vi "Drivetrain Manager.vi"(10 "setpoint":dbl) -> ()   [LabVIEW 2014]
uses:
  Robot Global Data.vi
  <vilib>/Rock Robotics/WPI/RobotDrive/WPI_RobotDriveGetSetRefNum.vi
  <vilib>/addons/control/pid/NI_PID_pid.lvlib
  <vilib>/addons/control/pid/pid.llb/PID (DBL).vi
panel:
  in  "PID gains":T1={"proportional gain (Kc)"=1.0, "integral time (Ti, min)"=0.01, "derivative time (Td, min)"=0.0} {"derivative time (Td, min)" format="%.3f"; "integral time (Ti, min)" format="%.3f"; "proportional gain (Kc)" format="%.3f"}
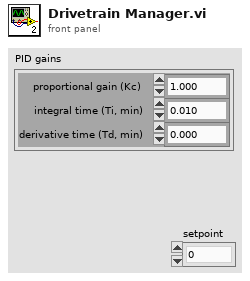
[diagram p1: front panel]
types:
  T1 = cluster{"proportional gain (Kc)":dbl, "integral time (Ti, min)":dbl, "derivative time (Td, min)":dbl}
  T2 = typedef "WPI_EncoderDevRef.ctl" = cluster{"DevStatus":errorcluster, "EncoderIndex":T3, "CounterIndex":T4, "DistancePerCount":dbl, "Decoding Type":T5}
  T3 = typedef "FPGA_EncoderIdx.ctl" = enum8{"Enc 0", "Enc 1", "Enc 2", "Enc 3", "Enc 4", "Enc 5", "Enc 6", "Enc 7", "Invalid"}
  T4 = typedef "FPGA_CounterCtrSystemIndex.ctl" = enum8{"Ctr 0", "Ctr 1", "Ctr 2", "Ctr 3", "Ctr 4", "Ctr 5", "Ctr 6", "Ctr 7", "Invalid"}
  T5 = typedef "WPI_EncoderType.ctl" = enum16{"1x", "2x", "4x"}
  T6 = typedef "WPI_RobotDriveDevRef.ctl" = cluster{"DevStatus":errorcluster, "Motors[]":T7[], "Square Inputs":bool, "Max Output":dbl}
  T7 = typedef "WPI_MotorControlDeviceRef.ctl" = cluster{"DeviceStatus":errorcluster, "Type":T8, "PWM":cluster{"Controller":T9, "PWM Channel":T10, "DeadBand":T11}, "CAN":cluster{"Device Number":u8, "Control Mode":T12, "Semaphore":T13, "Max Vout":dbl, "TalonSRX Control Mode":T14}, "Invert":bool, "TransformRef":T15, "InvTransformRef":T15}
  T8 = typedef "WPI_MotorControlType.ctl" = enum16{"PWM", "CAN", "CANTalonSRX"}
  T9 = typedef "FPGA_TypedefDigitalModule.ctl" = enum16{"Controller 1"}
  T10 = typedef "FPGA_DIOPWMChannel.ctl" = enum8{"PWM 0", "PWM 1", "PWM 2", "PWM 3", "PWM 4", "PWM 5", "PWM 6", "PWM 7", "PWM 8", "PWM 9", "PWM MXP 0", "PWM MXP 1", "PWM MXP 2", "PWM MXP 3", "PWM MXP 4", "PWM MXP 5", "PWM MXP 6", "PWM MXP 7", "PWM MXP 8", "PWM MXP 9", "Invalid"}
  T11 = typedef "WPI_PWMDeadband.ctl" = cluster{"Name":string, "maxPositivePwm":i32, "minPositivePwm":i32, "centerPwm":i32, "maxNegativePwm":i32, "minNegativePwm":i32, "angularRange":u16}
  T12 = typedef "WPI_CANJaguar_ControlMode.ctl" = enum8{"Percent VBus", "Current", "Speed", "Position", "Voltage"}
  T13 = typedef "Semaphore RefNum" = refnum<k1>
  T14 = typedef "WPI_CANTalonSRX_APIControlMode.ctl" = enum8{"Percent VBus", "Speed", "Position", "Slave", "Unchanged / Invalid"}
  T15 = typedef "WPI_PWMTransform_ConPane.ctl" = refnum<vi>
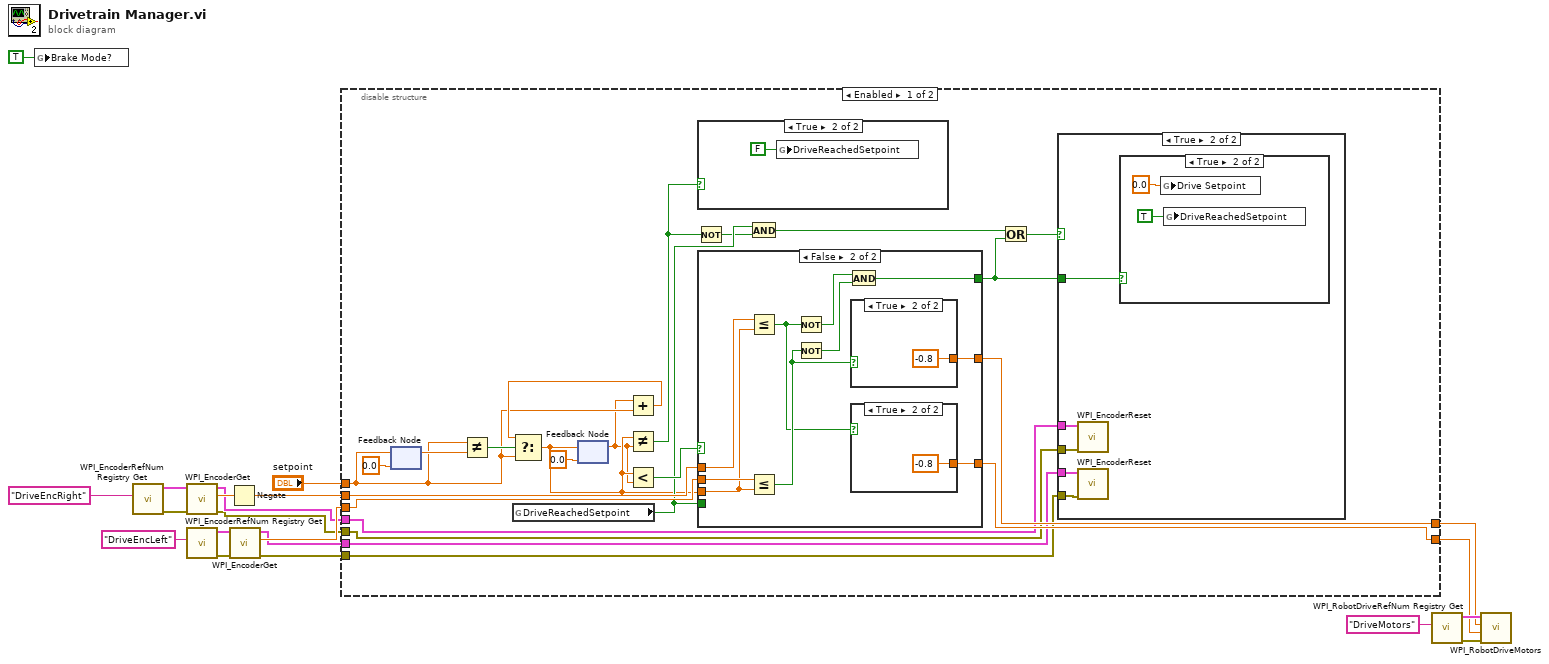
[diagram p0: block diagram]
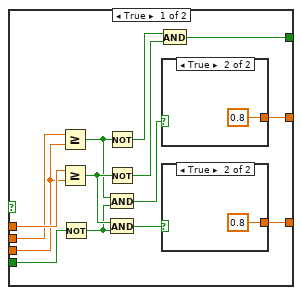
[diagram p5: hidden frame]
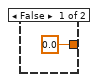
[diagram p6: hidden frame]
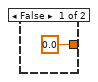
[diagram p7: hidden frame]
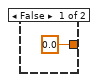
[diagram p8: hidden frame]
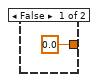
[diagram p9: hidden frame]
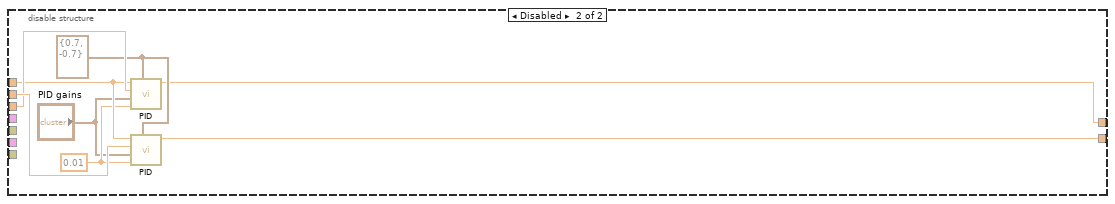
[diagram p10: hidden frame]
diagram:
  n1 = global write "Robot Global Data.vi" "Brake Mode?"(TRUE) -> ()
  n2 = call <vilib>:"WPI_EncoderRefNum Registry Get.vi"("refnum name"="DriveEncRight") -> ("error out"=w13:errorcluster, "EncoderDevRef"=w14:T2)  [unwired: 9 in]
  n3 = call <vilib>:"WPI_EncoderGet.vi"("error in (no error)"=w13, "EncoderDevRef"=w14) -> ("error out"=w1:errorcluster, "Distance"=w6:dbl, "EncoderDevRef"=w2:T2)  [unwired: 4 in, 3 out]
  n4 = call <vilib>:"WPI_EncoderRefNum Registry Get.vi"("refnum name"="DriveEncLeft") -> ("error out"=w10:errorcluster, "EncoderDevRef"=w11:T2)  [unwired: 9 in]
  n5 = Negate(x=w6) -> (-x=w5:dbl)
  n6 = call <vilib>:"WPI_EncoderGet.vi"("error in (no error)"=w10, "EncoderDevRef"=w11) -> ("error out"=w3:errorcluster, "Distance"=w7:dbl, "EncoderDevRef"=w4:T2)  [unwired: 4 in, 3 out]
  n7 = disable-structure shown="Enabled" {
    disable-tunnel: [w42 w85] -> w16
    disable-tunnel: [w41 w86] -> w15
    disable-tunnel: "setpoint" -> [w23 w89]
    disable-tunnel: w7 -> [w40 w90]
    disable-tunnel: w5 -> [w39 w91]
    disable-tunnel: w4 -> [w35 _]
    disable-tunnel: w3 -> [w36 _]
    disable-tunnel: w2 -> [w37 _]
    disable-tunnel: w1 -> [w38 _]
    frame Enabled {
      n8 = feedback #1(0.0 ("setpoint")) -> (w26:dbl)
      n9 = feedback-in #1(w23) -> ()
      n10 = Not Equal?(x=w23, y=w26) -> (x != y?=w25:bool)
      n11 = global read "Robot Global Data.vi" "DriveReachedSetpoint"() -> (w34:bool)
      n12 = feedback #2(0.0 ("setpoint")) -> (w21:dbl)
      n13 = Add(x=w21, y=w23) -> (x+y=w24:dbl)
      n14 = Select(t=w24, s=w25, f=w23) -> (s? t:f=w22:dbl)
      n15 = feedback-in #2(w22) -> ()
      n16 = Not Equal?(x=w22, y=w21) -> (x != y?=w29:bool)
      n17 = Less?(x=w22, y=w21) -> (x < y?=w43:bool)
      n18 = Not(x=w29) -> (.not. x?=w30:bool)
      n19 = case shown="True" w29 {
        frame False {
        }
        frame True {
          n20 = global write "Robot Global Data.vi" "DriveReachedSetpoint"(FALSE) -> ()
        }
      }
      n21 = case shown="False" w43 {
        tunnel: w39 -> [w65 w79]
        tunnel: w40 -> [w64 w78]
        tunnel: w22 -> [w63 w77]
        tunnel: [w61 w76] -> w41
        tunnel: [w62 w75] -> w42
        tunnel: [w58 w73] -> w33
        tunnel: w34 -> [w54 _]
        frame True {
          n22 = Greater Or Equal?(x=w64, y=w63) -> (x >= y?=w53:bool)
          n23 = Greater Or Equal?(x=w65, y=w63) -> (x >= y?=w56:bool)
          n24 = Not(x=w54) -> (.not. x?=w52:bool)
          n25 = Not(x=w53) -> (.not. x?=w60:bool)
          n26 = Not(x=w56) -> (.not. x?=w59:bool)
          n27 = And(x=w53, y=w52) -> (x .and. y?=w55:bool)
          n28 = And(x=w56, y=w52) -> (x .and. y?=w57:bool)
          n29 = And(x=w60, y=w59) -> (x .and. y?=w58:bool)
          n30 = case shown="True" w55 {
            tunnel: [0.0 0.8] -> w62
            frame False {
            }
            frame True {
            }
          }
          n31 = case shown="True" w57 {
            tunnel: [0.0 0.8] -> w61
            frame False {
            }
            frame True {
            }
          }
        }
        frame False {
          n32 = Less Or Equal?(x=w79, y=w77) -> (x <= y?=w70:bool)
          n33 = Less Or Equal?(x=w78, y=w77) -> (x <= y?=w71:bool)
          n34 = Not(x=w70) -> (.not. x?=w74:bool)
          n35 = Not(x=w71) -> (.not. x?=w72:bool)
          n36 = And(x=w74, y=w72) -> (x .and. y?=w73:bool)
          n37 = case shown="True" w71 {
            tunnel: [0.0 -0.8] -> w75
            frame False {
            }
            frame True {
            }
          }
          n38 = case shown="True" w70 {
            tunnel: [0.0 -0.8] -> w76
            frame False {
            }
            frame True {
            }
          }
        }
      }
      n39 = And(x=w34, y=w30) -> (x .and. y?=w32:bool)
      n40 = Or(x=w32, y=w33) -> (x .or. y?=w31:bool)
      n41 = case shown="True" w31 {
        tunnel: w38 -> [_ w46]
        tunnel: w37 -> [_ w47]
        tunnel: w36 -> [_ w49]
        tunnel: w35 -> [_ w48]
        tunnel: w33 -> [_ w45]
        frame False {
        }
        frame True {
          n42 = call <vilib>:"WPI_EncoderReset.vi"("error in (no error)"=w46, "EncoderDevRef"=w47) -> ()  [unwired: 8 in, 2 out]
          n43 = call <vilib>:"WPI_EncoderReset.vi"("error in (no error)"=w49, "EncoderDevRef"=w48) -> ()  [unwired: 8 in, 2 out]
          n44 = case shown="True" w45 {
            frame False {
            }
            frame True {
              n45 = global write "Robot Global Data.vi" "Drive Setpoint"(0.0) -> ()
              n46 = global write "Robot Global Data.vi" "DriveReachedSetpoint"(TRUE) -> ()
            }
          }
        }
      }
    }
    frame Disabled {
      w87 = cluster{"output high":dbl, "output low":dbl} {"output high"=0.7, "output low"=-0.7} ("output range")
      w88 = 0.01
      n47 = call-poly <vilib>:"PID.vi"("output range"=w87, "dt (s)"=w88, "PID gains"="PID gains", "process variable"=w90, "setpoint"=w89) -> ("output"=w85:dbl)  [unwired: 5 in, 1 out]
      n48 = call-poly <vilib>:"PID.vi"("output range"=w87, "dt (s)"=w88, "PID gains"="PID gains", "process variable"=w91, "setpoint"=w89) -> ("output"=w86:dbl)  [unwired: 5 in, 1 out]
    }
  }
  n49 = call <vilib>:"WPI_RobotDriveRefNum Registry Get.vi"("refnum name"="DriveMotors") -> ("error out"=w17:errorcluster, "RobotDriveDevRef"=w18:T6)  [unwired: 9 in]
  n50 = call <vilib>:"WPI_RobotDriveMotors.vi"("error in (no error)"=w17, "RightSpeed"=w15, "LeftSpeed"=w16, "RobotDriveDevRef"=w18) -> ()  [unwired: 5 in, 3 out]
